vi "Corr Transducers Fill ADC Channel Lists.vi"(8 "error in":errorcluster, 10 "digitizer channels count (0)":i32, 11 "transducer list ref":refnum<vi>) -> (0 "error out":errorcluster, 3 "transducer list ref out":refnum<vi>)   [LabVIEW 2018]
doc: "Fills the digitizers channels list in the transducers list. Note the transducers array MUST be unlinked from typedef!"
uses:
  Corr Tranducer ADC Channel.ctl
panel:
  in  "Ring":T1
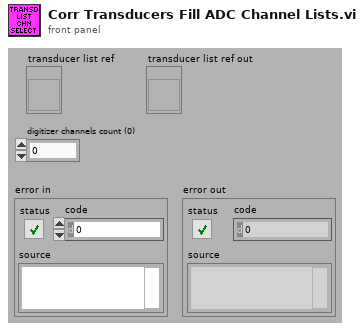
[diagram p1: front panel]
types:
  T1 = typedef "Corr Tranducer ADC Channel.ctl" = u16
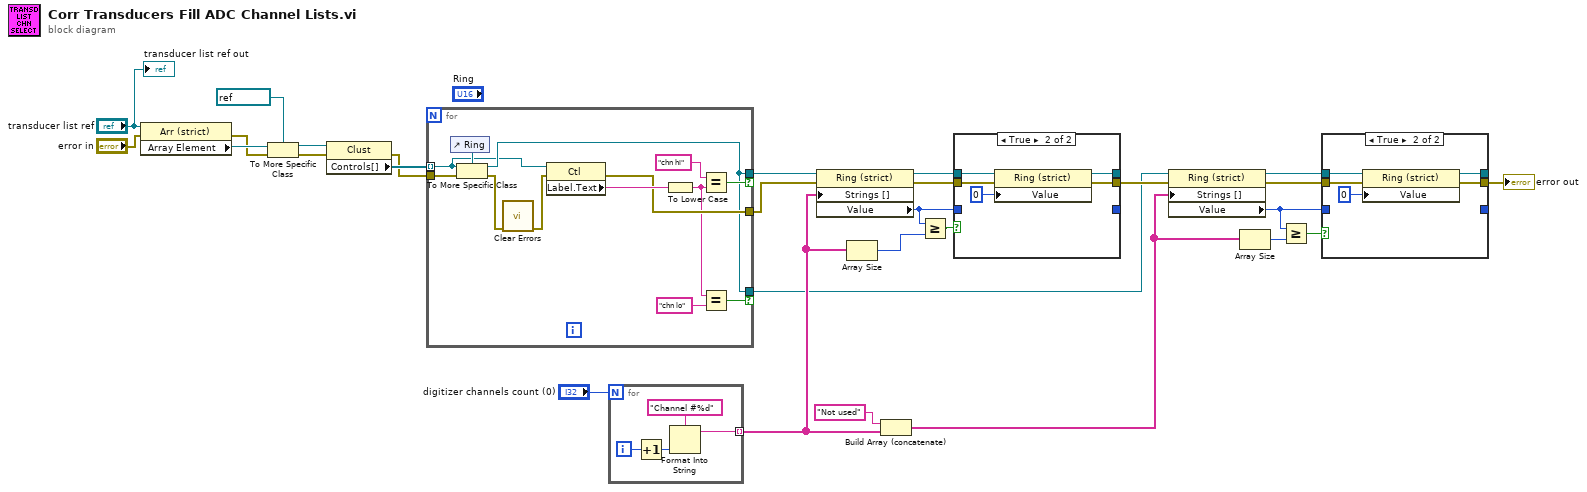
[diagram p0: block diagram]
diagram:
  n1 = property class="Arr (strict)"(reference="transducer list ref", error in="error in") -> (error out=w27:errorcluster, "Array Element"=w28:refnum<vi>)  [unwired: 1 out]
  n2 = To More Specific Class(target class=refnum<vi> refnum ("Cluster"), reference=w28, error in=w27) -> (specific class reference=w25:refnum<vi>, error out=w26:errorcluster)
  n3 = property class="Clust"(reference=w25, error in=w26) -> (error out=w21:errorcluster, "Controls[]"=w24:refnum<vi>[])  [unwired: 1 out]
  n4 = for {
    tunnel: w24 -> [w31] mode=indexing
    tunnel: [w33] -> w4 if=w36
    tunnel: [w39] -> w5
    tunnel: w21 -> [w34]
    tunnel: [w33] -> w6 if=w35
    n5 = control-ref of="Ring"() -> (w32:refnum<vi>)
    n6 = To More Specific Class(target class=w32, reference=w31, error in=w34) -> (specific class reference=w33:refnum<vi>, error out=w30:errorcluster)
    n7 = call <vilib>:"Clear Errors.vi"("error in (no error)"=w30) -> ("error out"=w29:errorcluster)  [unwired: 5 in, 1 out]
    n8 = property class="Ctl"(reference=w31, error in=w29) -> (error out=w39:errorcluster, "Label.Text"=w40:string)  [unwired: 1 out]
    n9 = To Lower Case(string=w40) -> (all lower case string=w38:string)
    n10 = Equal?(x="chn hi", y=w38) -> (x = y?=w36:bool)
    n11 = Equal?(x=w38, y="chn lo") -> (x = y?=w35:bool)
  }
  n12 = for {
    N: "digitizer channels count (0)" -> [_]
    tunnel: [w44] -> w14 mode=indexing
    i -> [w43]
    n13 = Increment(x=w43) -> (x+1=w42:i32)
    n14 = Format Into String(format string="Channel #%d", w42) -> (resulting string=w44:string)  [unwired: 2 in, 1 out]
  }
  n15 = property class="Ring (strict)"(reference=w4, error in=w5, "Strings []"=w14) -> (reference out=w18:refnum<vi>, error out=w19:errorcluster, "Value"=w16:T1)
  n16 = Array Size(array=w14) -> (size(s)=w20:i32)
  n17 = Build Array (concatenate)("Not used" ("y"), w14) -> (w11:string[])
  n18 = Greater Or Equal?(x=w16, y=w20) -> (x >= y?=w17:bool)
  n19 = case shown="True" w17 {
    tunnel: w19 -> [w48 w53]
    tunnel: w18 -> [w47 w52]
    tunnel: [w48 w50] -> w15
    tunnel: [w47 w49] -> _
    tunnel: w16 -> [w46 _]
    tunnel: [w46 _] -> _
    frame False {
    }
    frame True {
      n20 = property class="Ring (strict)"(reference=w52, error in=w53, "Value"=u16 0) -> (reference out=w49:refnum<vi>, error out=w50:errorcluster)
    }
  }
  n21 = property class="Ring (strict)"(reference=w6, error in=w15, "Strings []"=w11) -> (reference out=w9:refnum<vi>, error out=w10:errorcluster, "Value"=w7:T1)
  n22 = Array Size(array=w11) -> (size(s)=w12:i32)
  n23 = Greater Or Equal?(x=w7, y=w12) -> (x >= y?=w8:bool)
  n24 = case shown="True" w8 {
    tunnel: w10 -> [w56 w61]
    tunnel: w9 -> [w55 w60]
    tunnel: [w56 w58] -> w1
    tunnel: [w55 w57] -> _
    tunnel: w7 -> [w54 _]
    tunnel: [w54 _] -> _
    frame False {
    }
    frame True {
      n25 = property class="Ring (strict)"(reference=w60, error in=w61, "Value"=u16 0) -> (reference out=w57:refnum<vi>, error out=w58:errorcluster)
    }
  }
  "error out" <- w1
  "transducer list ref out" <- "transducer list ref"
